vi "Write Error Pointer.vi"(8 "error in (no error)":errorcluster, 10 "error":errorcluster, 11 "Error Pointer in":refnum<class "Error Pointer.lvclass">) -> (0 "error out":errorcluster, 3 "Error Pointer in":refnum<class "Error Pointer.lvclass">)   [LabVIEW 2019, in "DSF Core.lvlib" / "Error Pointer.lvclass"]
uses:
  Error Pointer.lvclass
  C:/Program Files (x86)/National Instruments/LabVIEW 2019/vi.lib/NI/Memory Manager/Classes/Pointer/Pointer.lvclass
  <vilib>/NI/Memory Manager/Classes/Pointer/Pointer.lvclass/Pointer.ctl
  <vilib>/NI/Memory Manager/Classes/Pointer/Write 1D U8.vi
  <vilib>/NI/Memory Manager/Classes/Pointer/Write (No Check).vi
  <vilib>/NI/Memory Manager/Classes/Pointer/Write (No Check) 1D U8.vi
  <vilib>/NI/Memory Manager/Classes/Pointer/Check Move.vi
  <vilib>/NI/Memory Manager/Classes/Pointer/Check Null Pointer.vi
  <vilib>/NI/Memory Manager/Classes/Pointer/Clear (No Check).vi
  <vilib>/NI/Memory Manager/Classes/Pointer/Check Length.vi
  <vilib>/NI/Memory Manager/Classes/Pointer/Get Address.vi
  <vilib>/NI/Memory Manager/Classes/Pointer/Check Count.vi
  <vilib>/NI/Memory Manager/Classes/Pointer/Check Bounds (Power of 2).vi
  <vilib>/NI/Memory Manager/Classes/Pointer/Errors.vi
  <vilib>/NI/Memory Manager/Classes/Pointer/Null Pointer.vi
  <vilib>/NI/Memory Manager/Classes/Pointer/Is Null.vi
  <vilib>/NI/Memory Manager/Classes/Pointer/Get Size.vi
  <vilib>/NI/Memory Manager/Classes/Pointer/Check Bounds (Pointer).vi
  <vilib>/NI/Memory Manager/Classes/Pointer/Out of Bounds.vi
  <vilib>/NI/Memory Manager/Classes/Pointer/Check Bounds.vi
  <vilib>/NI/Memory Manager/Classes/Pointer/Create Error.vi
  <vilib>/NI/Memory Manager/VIs/Write String to Source.vi
  <vilib>/NI/Memory Manager/Classes/Pointer/Write Pointer Size to Error.vi
  <vilib>/NI/Memory Manager/VIs/Write Numeric to Source.vi
  <vilib>/NI/Memory Manager/VIs/Write Numeric Scalar to Source (Base10 U64).vi
  <vilib>/NI/Memory Manager/Classes/Pointer/Check Bounds (Buffer).vi
  <vilib>/NI/Memory Manager/VIs/New Error Cluster.vi
  <vilib>/NI/Memory Manager/VIs/New Error Cluster (512B).vi
  <vilib>/NI/Memory Manager/VIs/Set Error Status.vi
  <vilib>/NI/Memory Manager/VIs/Set Error Code.vi
  <vilib>/NI/Memory Manager/VIs/Set Error Source.vi
  <vilib>/NI/Memory Manager/Constants/Constants.vi
  <vilib>/NI/Memory Manager/Constants/Library Name.vi
  <vilib>/NI/Memory Manager/Classes/Pointer/Pointer Error Info.vi
  <vilib>/NI/Memory Manager/Constants/Pointer Class Name.vi
  <vilib>/NI/Memory Manager/Classes/Pointer/Buffer Underflow.vi
  <vilib>/NI/Memory Manager/Classes/Pointer/Pointer.lvclass
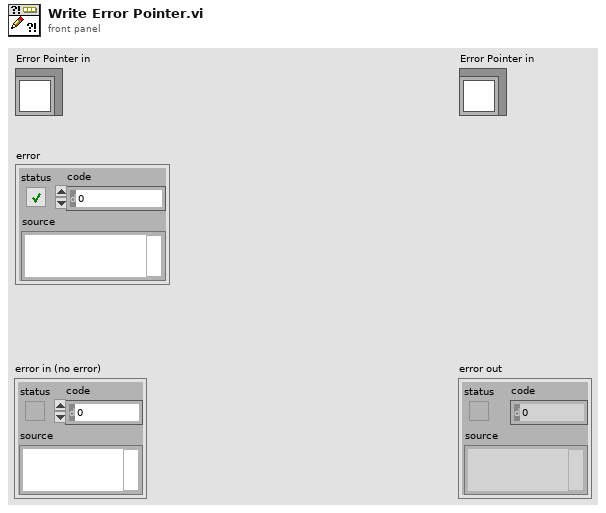
[diagram p1: front panel]
types:
  T1 = enum16{"big-endian, network order", "native, host order", "little-endian"}
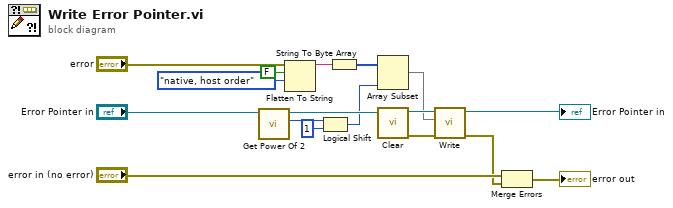
[diagram p0: block diagram]
diagram:
  n1 = call "Get Power Of 2.vi"("Error Pointer in"="Error Pointer in") -> ("power of 2"=w3:i16, "Error Pointer out"=w4:refnum<class "Error Pointer.lvclass">)  [unwired: 9 in]
  n2 = Flatten To String(anything="error", prepend array or string size? (T)=FALSE, byte order (0:big-endian, network order)=T1."native, host order") -> (data string=w14:string)  [unwired: 1 in, 2 out]
  n3 = Logical Shift(y=w3, x=i64 1) -> (x << y=w1:i64)
  n4 = String To Byte Array(string=w14) -> (unsigned byte array=w12:u8[])
  n5 = Array Subset(array=w12, length=w1) -> (w11:u8[])  [unwired: 1 in]
  n6 = call <vilib>:"Clear.vi"("Pointer in"=w4) -> ("error out"=w10:errorcluster, "Pointer out"=w13:refnum<class "Error Pointer.lvclass">)  [unwired: 9 in]
  n7 = call-poly <vilib>:"Write.vi"("error in (no error)"=w10, "buffer in"=w11, "Pointer in"=w13) -> ("error out"=w7:errorcluster, "Pointer out"=→"Error Pointer in":refnum<class "Error Pointer.lvclass">)  [unwired: 5 in, 2 out]
  n8 = Merge Errors("error in (no error)", w7) -> (→"error out":errorcluster)
